vi "4 byte data to number.vi"(0 "4":u8, 1 "3":u8, 2 "2":u8, 3 "1":u8) -> (5 "data out":dbl)   [LabVIEW 2013]
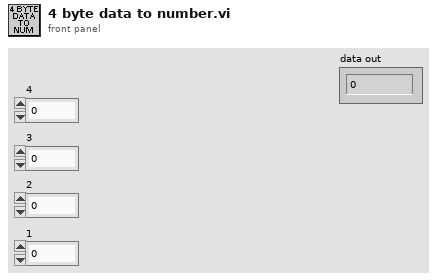
[diagram p1: front panel]
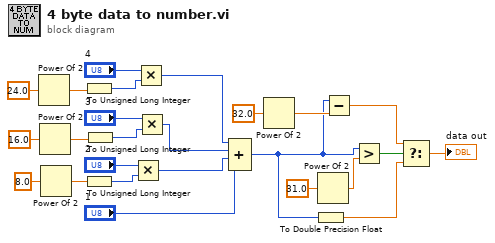
[diagram p0: block diagram]
diagram:
  n1 = Power Of 2(x=24.0) -> (2^x=w21:dbl)
  n2 = Power Of 2(x=16.0) -> (2^x=w19:dbl)
  n3 = Power Of 2(x=8.0) -> (2^x=w15:dbl)
  n4 = To Unsigned Long Integer(number=w21) -> (unsigned 32bit integer=w22:u32)
  n5 = To Unsigned Long Integer(number=w15) -> (unsigned 32bit integer=w14:u32)
  n6 = To Unsigned Long Integer(number=w19) -> (unsigned 32bit integer=w18:u32)
  n7 = Multiply(x="2", y=w14) -> (x*y=w11:u32)
  n8 = Multiply(x="4", y=w22) -> (x*y=w13:u32)
  n9 = Multiply(x="3", y=w18) -> (x*y=w12:u32)
  n10 = Compound Arithmetic op=ADD(w13, w12, w11, "1") -> (w3:u32)
  n11 = Power Of 2(x=32.0) -> (2^x=w6:dbl)
  n12 = To Double Precision Float(number=w3) -> (double precision float=w2:dbl)
  n13 = Power Of 2(x=31.0) -> (2^x=w9:dbl)
  n14 = Subtract(x=w3, y=w6) -> (x-y=w5:dbl)
  n15 = Greater?(x=w3, y=w9) -> (0:w8:bool)
  n16 = Select(t=w5, s=w8, f=w2) -> (s? t:f=→"data out":dbl)
